vi "CreateQueues.vi"(9 "create if not found? (T)":bool=TRUE, 10 "client configuration":T2) -> (3 "output cluster":T1)   [LabVIEW 2014]
uses:
  typedefs/clientConfiguration.ctl
  typedefs/clientStatus.ctl
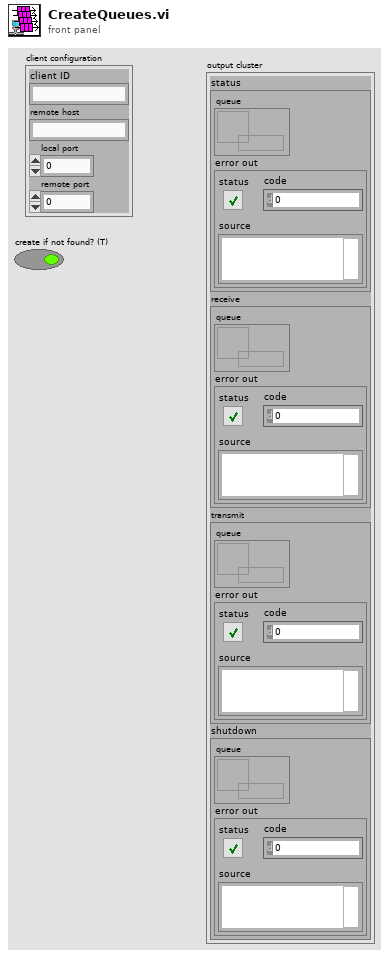
[diagram p1: front panel]
types:
  T1 = cluster{"status":cluster{"queue":refnum<queue>, "error out":errorcluster}, "receive":cluster{"queue":refnum<queue>, "error out":errorcluster}, "transmit":cluster{"queue":refnum<queue>, "error out":errorcluster}, "shutdown":cluster{"queue":refnum<queue>, "error out":errorcluster}}
  T2 = typedef "clientConfiguration.ctl" = cluster{"client ID":string, "remote host":string, "local port":u16, "remote port":u16}
  T3 = cluster{"queue out":refnum<queue>, "error out":errorcluster}
  T4 = typedef "clientStatus.ctl" = cluster{"connected":bool, "sent":bool}
  T5 = cluster{"status":cluster{"queue out":refnum<queue>, "error out":errorcluster}, "receive":cluster{"queue out":refnum<queue>, "error out":errorcluster}, "transmit":cluster{"queue out":refnum<queue>, "error out":errorcluster}, "shutdown":cluster{"queue out":refnum<queue>, "error out":errorcluster}}
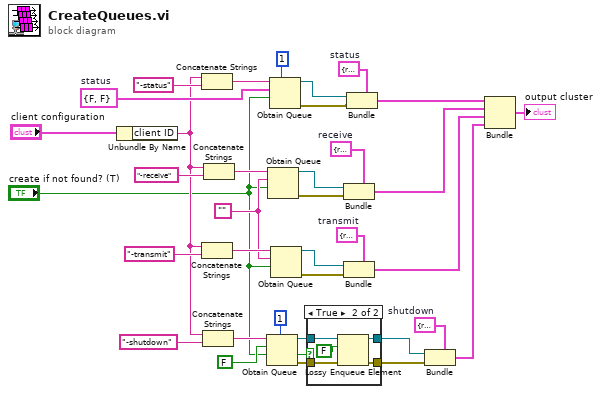
[diagram p0: block diagram]
diagram:
  w10 = T3 {"queue out"=refnum, "error out"={"status"=FALSE, "code"=0, "source"=""}}  # shutdown
  w12 = T3 {"queue out"=refnum, "error out"={"status"=FALSE, "code"=0, "source"=""}}  # transmit
  w15 = T3 {"queue out"=refnum, "error out"={"status"=FALSE, "code"=0, "source"=""}}  # receive
  w19 = T3 {"queue out"=refnum, "error out"={"status"=FALSE, "code"=0, "source"=""}}  # status
  w24 = T4 {"connected"=FALSE, "sent"=FALSE}  # status
  w28 = ""
  n1 = Unbundle By Name("client configuration") -> ("client ID"=w23:string)
  n2 = Concatenate Strings(w23, "-status" ("string")) -> (w34:string)
  n3 = Concatenate Strings(w23, "-transmit" ("string")) -> (w31:string)
  n4 = Concatenate Strings(w23, "-shutdown" ("string")) -> (w36:string)
  n5 = Concatenate Strings(w23, "-receive" ("string")) -> (w29:string)
  n6 = Obtain Queue(max queue size (-1, unlimited)=1, name (unnamed)=w36, element data type=FALSE, create if not found? (T)="create if not found? (T)") -> (queue out=w11:refnum<queue>, created new?=w1:bool, error out=w3:errorcluster)  [unwired: 1 in]
  n7 = Obtain Queue(name (unnamed)=w29, element data type=w28, create if not found? (T)="create if not found? (T)") -> (queue out=w17:refnum<queue>, error out=w16:errorcluster)  [unwired: 2 in, 1 out]
  n8 = Obtain Queue(max queue size (-1, unlimited)=1, name (unnamed)=w34, element data type=w24, create if not found? (T)="create if not found? (T)") -> (queue out=w20:refnum<queue>, error out=w21:errorcluster)  [unwired: 1 in, 1 out]
  n9 = Obtain Queue(name (unnamed)=w31, element data type=w28, create if not found? (T)="create if not found? (T)") -> (queue out=w14:refnum<queue>, error out=w13:errorcluster)  [unwired: 2 in, 1 out]
  n10 = case shown="True" w1 {
    tunnel: w11 -> [w38 w43]
    tunnel: [w38 w42] -> w4
    tunnel: w3 -> [w37 w41]
    tunnel: [w37 w40] -> w2
    frame False {
    }
    frame True {
      n11 = Lossy Enqueue Element(queue=w43, element=FALSE, error in (no error)=w41) -> (queue out=w42:refnum<queue>, error out=w40:errorcluster)  [unwired: 2 out]
    }
  }
  n12 = Bundle(cluster=w15, "queue out"=w17, "error out"=w16) -> (w9:T3)
  n13 = Bundle(cluster=w12, "queue out"=w14, "error out"=w13) -> (w8:T3)
  n14 = Bundle(cluster=w19, "queue out"=w20, "error out"=w21) -> (w18:T3)
  n15 = Bundle(cluster=w10, "queue out"=w4, "error out"=w2) -> (w7:T3)
  n16 = Bundle("status"=w18, "receive"=w9, "transmit"=w8, "shutdown"=w7) -> (→"output cluster":T5)  [unwired: 1 in]
